vi "crea vector de resolución.vi"(10 "Resolución":dbl) -> (2 "Vector resolución (r)":dbl[](array[numeric]))   [LabVIEW 2025]
doc: "Este VI crea el vector de resolución de 0 hasta el valor de resolución especificado por el usuario. La resolución se refiere al número de puntos por el que estará compuesta la gráfica."
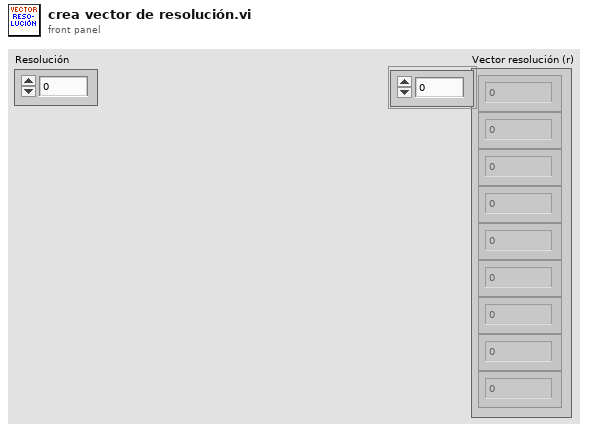
[diagram p1: front panel]
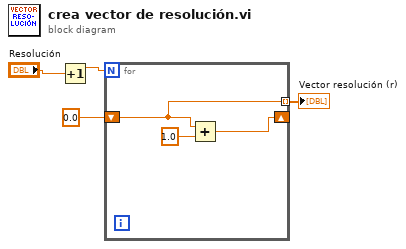
[diagram p0: block diagram]
diagram:
  n1 = Increment(x="Resolución") -> (x+1=w3:dbl)
  n2 = for {
    N: w3 -> [_]
    shift-right: [w6] -> _
    shift-left: 0.0 -> [w5]
    tunnel: [w5] -> w1 mode=indexing
    n3 = Add(x=w5, y=1.0) -> (x+y=w6:dbl)
  }
  "Vector resolución (r)" <- w1
